vi "Generate Simulated Data.vi"(8 "error in (no error)":errorcluster, 11 "Signal Type":T1 items=["Simulated", "Tektronics DPO2k/3k/4k", "PicoScope 2000a Series", "Keithley DMM7510", "PicoScope 5000a Series", "Arduino"]) -> (0 "error out":errorcluster, 2 "Graph Data":waveform(dbl)[](array[waveform]), 4 "Sampling time":dbl=0.001)   [LabVIEW 2017, in "Acquisition.lvlib"]
doc: "Generates sample waveforms according to the signal type in the HW Config input."
uses:
  Acquisition.lvlib
  Signal Type.ctl
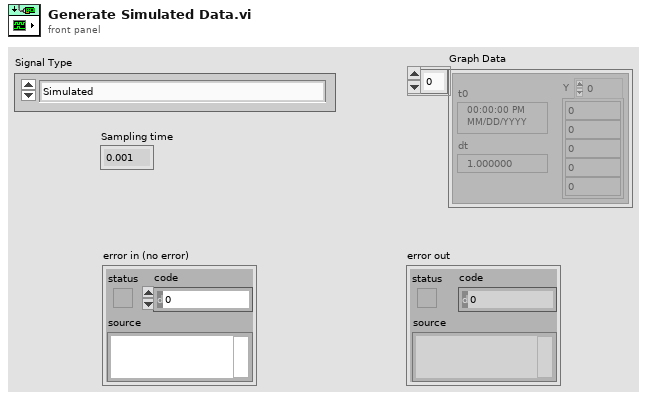
[diagram p1: front panel]
types:
  T1 = typedef "Acquisition.lvlib/Signal Type.ctl" = u16
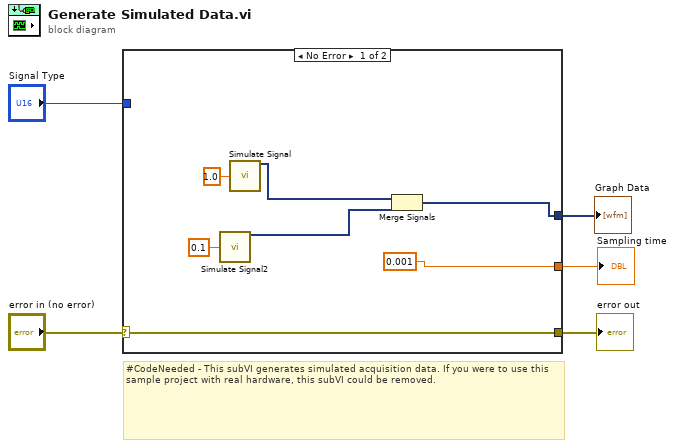
[diagram p0: block diagram]
diagram:
  # "#CodeNeeded - This subVI generates simulated acquisition data. If you were to use this sample project with real hardware, this subVI could be removed."
  n1 = case shown="No Error" "error in (no error)" {
    selector: "error in (no error)" -> [w12 w13]
    tunnel: [w12 w13] -> w4
    tunnel: [w10 _] -> w3
    tunnel: "Signal Type" -> [_ _]
    tunnel: [0.001 _] -> w1
    frame No Error {
      n2 = call "Simulate Signal2"("Amplitude"=0.1) -> ("Sine"=w9:dynamicdata)  [unwired: 13 in, 1 out]
      n3 = call "Simulate Signal"("Amplitude"=1.0) -> ("Sine"=w11:dynamicdata)  [unwired: 13 in, 1 out]
      n4 = Merge Signals(w11, w9) -> (w10:dynamicdata)
    }
    frame Error {
    }
  }
  "error out" <- w4
  "Graph Data" <- w3
  "Sampling time" <- w1
